vi "Refresh Possible Connections.vi"(8 "error in":errorcluster, 11 "slsc switch custom device in":T1 format="%.0x") -> (0 "error out":errorcluster, 3 "slsc switch custom device out":T1 format="%.0x")   [LabVIEW 2020, in "SLSC Switch Scripting.lvlib"]
uses:
  SLSC Switch Scripting.lvlib
  <vilib>/NI VeriStand/Custom Device API/Custom Device Item Ref.ctl
  Routing and Faulting/Routing and Faulting Hardware API/Routing and Faulting Hardware API.lvlib
  <vilib>/NI VeriStand/Custom Device API/Custom Device API.lvlib
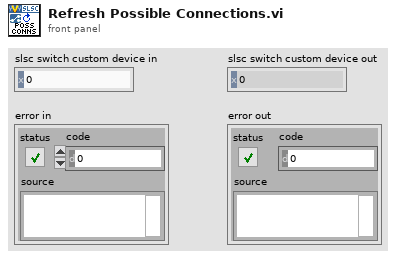
[diagram p1: front panel]
types:
  T1 = typedef "Custom Device API.lvlib/Custom Device Item Ref.ctl" = u64
  T2 = typedef "Routing and Faulting Hardware API.lvlib/Possible Connections for Endpoint.ctl" = cluster{"Source":string, "Destinations":string[]}
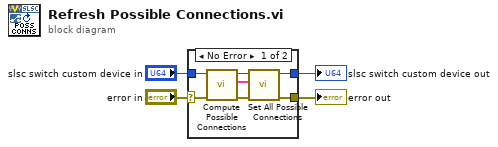
[diagram p0: block diagram]
diagram:
  n1 = case shown="No Error" "error in" {
    selector: "error in" -> [w9 w13]
    tunnel: [w11 w12] -> w4
    tunnel: "slsc switch custom device in" -> [w8 w12]
    tunnel: [w5 w13] -> w1
    frame No Error {
      n2 = call "Compute Possible Connections.vi"("error in"=w9, "slsc switch custom device in"=w8) -> ("error out"=w7:errorcluster, "possible connections"=w10:T2[], "slsc switch custom device out"=w6:T1)  [unwired: 7 in]
      n3 = call "Set All Possible Connections.vi"("error in (no error)"=w7, "Possible Connections"=w10, "Hardware Ref in"=w6) -> ("error out"=w5:errorcluster, "Hardware Ref out"=w11:T1)  [unwired: 7 in]
    }
    frame Error {
    }
  }
  "slsc switch custom device out" <- w4
  "error out" <- w1
